vi "PH_Numbers.Set Precision of Number.vi"(1 "Number":dbl) -> (0 "Precision":i16)   [LabVIEW 2014, in "PH_Common.lvlib"]
doc: "This VI gets the place after decimal point for setting the precision of numbers converted to strings."
uses:
  PH_Common.lvlib
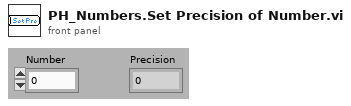
[diagram p1: front panel]
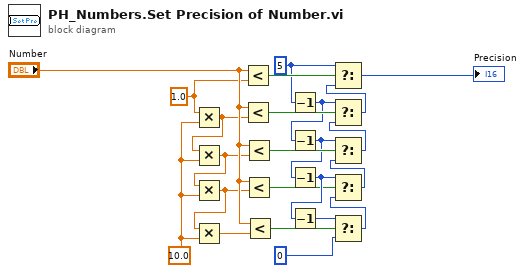
[diagram p0: block diagram]
diagram:
  w12 = 10.0 ("y")
  w16 = 1.0 ("y")
  w18 = i16 5 ("precision (6)")
  n1 = Multiply(x=w16, y=w12) -> (x*y=w15:dbl)
  n2 = Multiply(x=w15, y=w12) -> (x*y=w14:dbl)
  n3 = Multiply(x=w14, y=w12) -> (x*y=w11:dbl)
  n4 = Multiply(x=w11, y=w12) -> (x*y=w13:dbl)
  n5 = Less?(x="Number", y=w16) -> (x < y?=w20:bool)
  n6 = Less?(x="Number", y=w15) -> (x < y?=w19:bool)
  n7 = Less?(x="Number", y=w14) -> (x < y?=w8:bool)
  n8 = Less?(x="Number", y=w11) -> (x < y?=w5:bool)
  n9 = Less?(x="Number", y=w13) -> (x < y?=w4:bool)
  n10 = Decrement(x=w18) -> (x-1=w10:i16)
  n11 = Decrement(x=w10) -> (x-1=w3:i16)
  n12 = Decrement(x=w3) -> (x-1=w22:i16)
  n13 = Decrement(x=w22) -> (x-1=w2:i16)
  n14 = Select(t=w2, s=w4, f=i16 0) -> (s? t:f=w7:i16)
  n15 = Select(t=w22, s=w5, f=w7) -> (s? t:f=w6:i16)
  n16 = Select(t=w3, s=w8, f=w6) -> (s? t:f=w9:i16)
  n17 = Select(t=w10, s=w19, f=w9) -> (s? t:f=w17:i16)
  n18 = Select(t=w18, s=w20, f=w17) -> (s? t:f=→"Precision":i16)
